vi "MRC IMU Initialize.vi"(8 "error in (no error)":errorcluster) -> (0 "error out":errorcluster)   [LabVIEW 2026, in "MrcLib.lvlib"]
doc: "MRC_Status MRC_CALLCONV MRC_IMU_Initialize(void);"
uses:
  MrcLib.lvlib
  MrcLib.dll
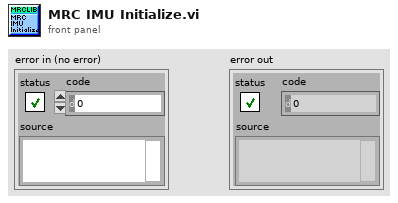
[diagram p1: front panel]
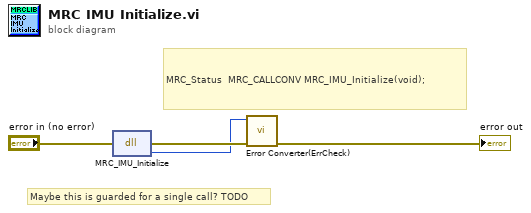
[diagram p0: block diagram]
diagram:
  # "Maybe this is guarded for a single call? TODO"
  # "MRC_Status  MRC_CALLCONV MRC_IMU_Initialize(void);"
  n1 = dll-call lib="MrcLib.*" fn="MRC_IMU_Initialize"(error in="error in (no error)") -> (error out=w3:errorcluster, w1:i32)  [unwired: 2 in, 1 out]
  n2 = call "Error Converter(ErrCheck).vi"("error in (no error)"=w3, "status"=w1) -> ("error out"=→"error out":errorcluster)  [unwired: 9 in]
